vi "test Deployment Import Configuration.vi"(8 "error in":errorcluster, 11 "TestCase in":refnum<class "Deployment.lvclass">) -> (0 "error out":errorcluster, 3 "TestCase out":refnum<class "Deployment.lvclass">)   [LabVIEW 2023, in "Deployment.lvclass"]
uses:
  Deployment.lvclass
  Deployment.lvclass/Deployment.ctl
  <vilib>/addons/_JKI Toolkits/VI Tester/TestCase.llb/TestCase.lvclass
  315b1c3a-44c8-49e8-b756-01f865c29b4a.vi
  <vilib>/NI/VeriStand Custom Device Testing Tools/VeriStandTestUtilities/VeriStandTestUtilities.lvlib
  Scripting/Ballard MIL-STD-1553 Scripting.lvlib
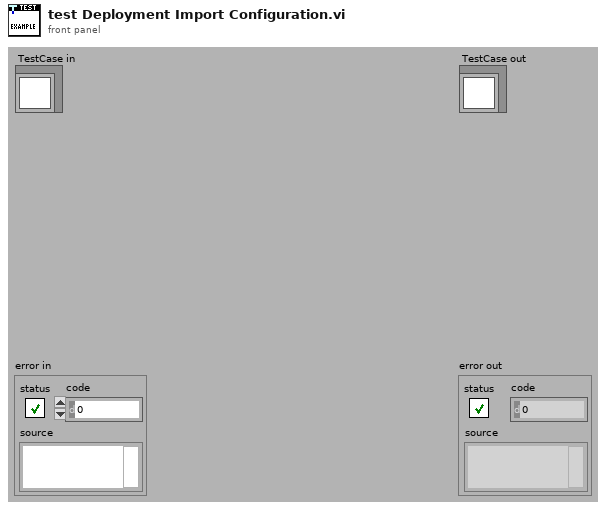
[diagram p1: front panel]
types:
  T1 = cluster{"Hardware File":path, "Parameters File":path}
  T2 = typedef "Custom Device API.lvlib/Custom Device Item Ref.ctl" = u64
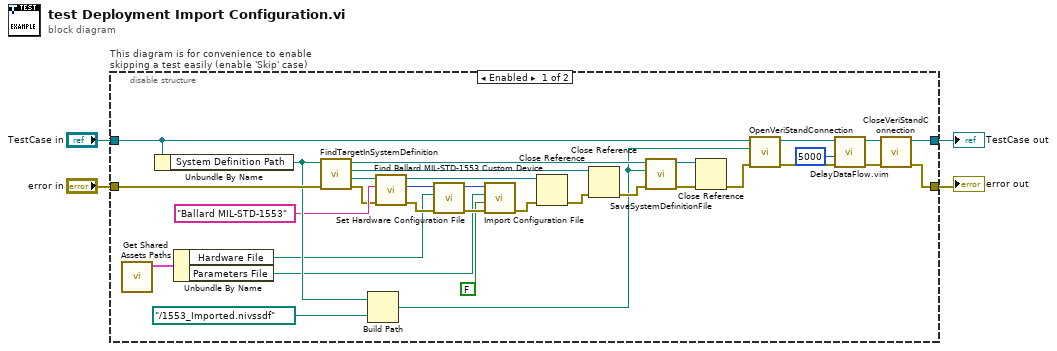
[diagram p0: block diagram]
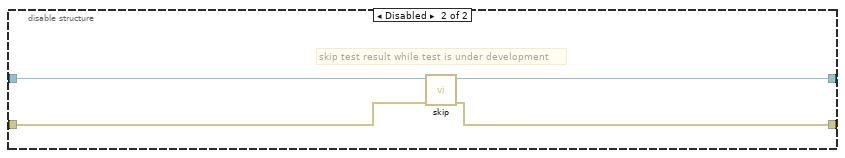
[diagram p2: hidden frame]
diagram:
  n1 = disable-structure "This diagram is for convenience to enable skipping a test easily (enable 'Skip' case)" shown="Enabled" {
    disable-tunnel: "TestCase in" -> [w29 w39]
    disable-tunnel: [w30 w37] -> w1
    disable-tunnel: [w32 w38] -> w3
    disable-tunnel: "error in" -> [w28 w36]
    frame Enabled {
      n2 = call "Get Shared Assets Paths.vi"() -> ("BC and RTs"=w8:T1)  [unwired: 9 in, 2 out]
      n3 = Unbundle By Name(w29) -> ("System Definition Path"=w26:path)
      n4 = Unbundle By Name(w8) -> ("Hardware File"=w7:path, "Parameters File"=w6:path)
      n5 = call <vilib>:"FindTargetInSystemDefinition.vi"("error in"=w28, "system definition path"=w26) -> ("error out"=w15:errorcluster, "Target"=w18:refnum<k24>, "Root"=w21:refnum<k24>, "System Definition"=w27:refnum<k24>)  [unwired: 6 in]
      n6 = Build Path(base path=w26, name or relative path=path "../1553_Imported.nivssdf") -> (appended path=w12:path)
      n7 = call "Find Ballard MIL-STD-1553 Custom Device.vi"("error in"=w15, "name"="Ballard MIL-STD-1553", "target in"=w18) -> ("error out"=w13:errorcluster, "Ballard MIL-STD 1553 custom device"=w14:T2, "target out"=w16:refnum<k24>)  [unwired: 5 in, 1 out]
      n8 = call "Set Hardware Configuration File.vi"("error in"=w13, "hardware configuration file path"=w7, "Ballard MIL-STD 1553 custom device in"=w14) -> ("error out"=w11:errorcluster, "Ballard MIL-STD 1553 custom device out"=w9:T2)  [unwired: 7 in]
      n9 = call "Import Configuration File.vi"("error in"=w11, "create Tx/Rx folders for subaddresses?"=FALSE, "parameters configuration file path"=w6, "Ballard MIL-STD 1553 custom device in"=w9) -> ("error out"=w10:errorcluster)  [unwired: 6 in, 1 out]
      n10 = Close Reference(reference=w16, error in (no error)=w10) -> (error out=w19:errorcluster)
      n11 = Close Reference(reference=w21, error in (no error)=w19) -> (error out=w20:errorcluster)
      n12 = call <vilib>:"SaveSystemDefinitionFile.vi"("error in (no error)"=w20, "System Definition File in"=w12, "System Definition Reference in"=w27) -> ("error out"=w23:errorcluster, "System Definition Reference out"=w24:refnum<k24>)  [unwired: 7 in]
      n13 = Close Reference(reference=w24, error in (no error)=w23) -> (error out=w22:errorcluster)
      n14 = call-dynamic "OpenVeriStandConnection.vi"("error in (no error)"=w22, "System Definition File"=w12, "VeriStand Test Case in"=w29) -> ("error out"=w35:errorcluster, "VeriStand Test Case out"=w31:refnum<class "Deployment.lvclass">)  [unwired: 6 in, 1 out]
      n15 = call "DelayDataFlow.vim"("value in"=w35, "milliseconds to wait"=u32 5000) -> ("value out"=w33:errorcluster)  [unwired: 2 in, 1 out]
      n16 = call-dynamic "CloseVeriStandConnection.vi"("error in (no error)"=w33, "VeriStand Test Case in"=w31) -> ("error out"=w32:errorcluster, "VeriStand Test Case out"=w30:refnum<class "Deployment.lvclass">)  [unwired: 8 in]
    }
    frame Disabled {
      # "skip test result while test is under development"
      n17 = call <vilib>:"skip.vi"("error in (no error)"=w36, "TestCase in"=w39) -> ("error out"=w38:errorcluster, "TestCase out"=w37:refnum<class "Deployment.lvclass">)  [unwired: 8 in]
    }
  }
  "error out" <- w3
  "TestCase out" <- w1
